vi "Fit Points to Circle.vi"(6 "Full Circle Plot":bool=TRUE, 8 "Error In":errorcluster, 9 "# Points (1000)":i32=1000, 10 "Y Array":dbl[](array[numeric]), 11 "X Array":dbl[](array[numeric])) -> (0 "Error Out":errorcluster, 3 "Fitted Circle Parameters":T1, 5 "Fitted Y Array":dbl[](array[numeric]), 7 "Fitted X Array":dbl[](array[numeric]))   [LabVIEW 2019]
uses:
  Fitted Circle Parameters.ctl
  <vilib>/Utility/error.llb/DialogType.ctl
  <vilib>/Utility/error.llb/Error Cluster From Error Code.vi
  <vilib>/ErrorRing/Error Ring.xnode
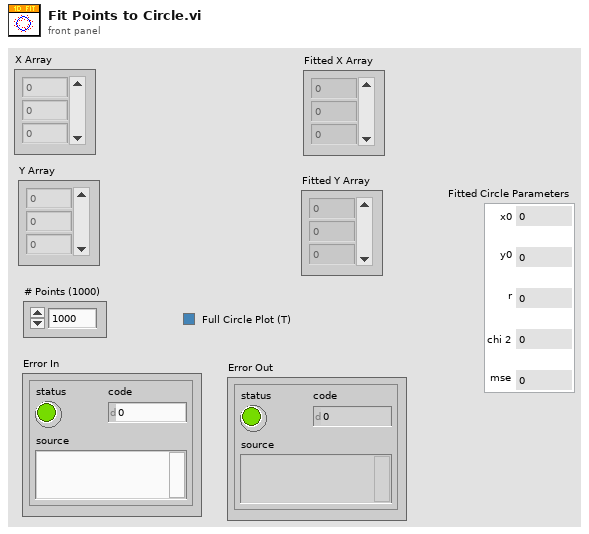
[diagram p1: front panel]
types:
  T1 = typedef "Fitted Circle Parameters.ctl" = cluster{"x0":dbl, "y0":dbl, "r":dbl, "chi 2":dbl, "mse":dbl}
  T2 = typedef "DialogType.ctl" = u16
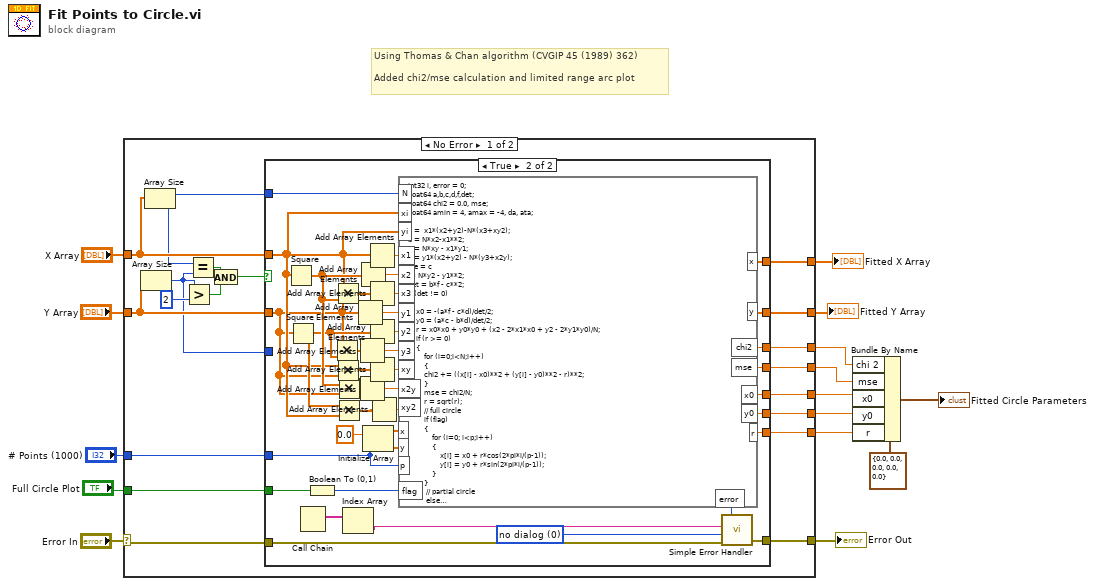
[diagram p0: block diagram]
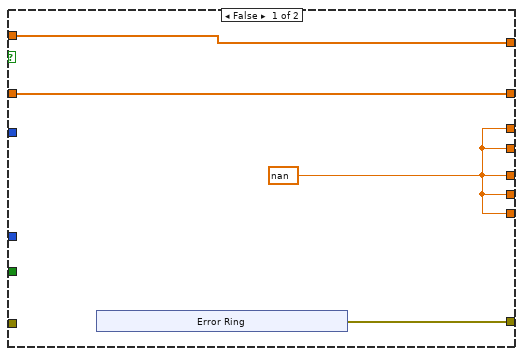
[diagram p2: hidden frame]
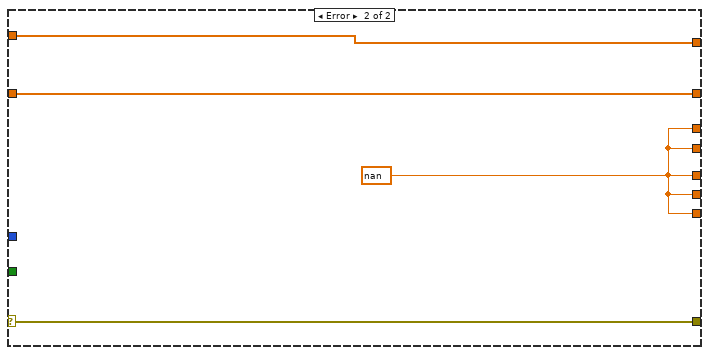
[diagram p3: hidden frame]
diagram:
  # "Using Thomas & Chan algorithm (CVGIP 45 (1989) 362)\n\nAdded chi2/mse calculation and limited range arc plot"
  n1 = case shown="No Error" "Error In" {
    selector: "Error In" -> [w20 w83]
    tunnel: "X Array" -> [w34 w82]
    tunnel: "Y Array" -> [w33 w81]
    tunnel: [w21 w83] -> w12
    tunnel: [w26 w82] -> w11
    tunnel: [w25 w81] -> w10
    tunnel: "# Points (1000)" -> [w27 _]
    tunnel: [w24 w80] -> w6
    tunnel: [w23 w80] -> w7
    tunnel: [w22 w80] -> w8
    tunnel: [w18 w80] -> w4
    tunnel: [w17 w80] -> w5
    tunnel: "Full Circle Plot" -> [w16 _]
    frame No Error {
      n2 = Array Size(array=w33) -> (size(s)=w28:i32)
      n3 = Array Size(array=w34) -> (size(s)=w19:i32)
      n4 = Greater?(x=w28, y=2) -> (0:w31:bool)
      n5 = Equal?(x=w19, y=w28) -> (x = y?=w30:bool)
      n6 = And(x=w30, y=w31) -> (x .and. y?=w29:bool)
      n7 = case shown="True" w29 {
        tunnel: w34 -> [w37 w44]
        tunnel: w33 -> [w36 w43]
        tunnel: w28 -> [_ _]
        tunnel: w27 -> [_ w49]
        tunnel: [w37 w77] -> w26
        tunnel: [w36 w76] -> w25
        tunnel: [w35 w75] -> w24
        tunnel: [w35 w74] -> w23
        tunnel: [w35 w73] -> w22
        tunnel: [w38 w56] -> w21
        tunnel: w20 -> [_ w55]
        tunnel: w19 -> [_ w50]
        tunnel: [w35 w48] -> w18
        tunnel: [w35 w47] -> w17
        tunnel: w16 -> [_ w46]
        frame False {
          w35 = nan ("x0")
          n8 = xnode "Error Ring"() -> ("error out"=w38:errorcluster)
        }
        frame True {
          w51 = T2 0 items=["no dialog", "OK message", "continue or stop message", "OK message + warnings", "continue/stop + warnings"] ("type of dialog (OK msg:1)")
          n9 = Square(x=w44) -> (x^2=w62:dbl[])
          n10 = Square(x=w43) -> (x^2=w59:dbl[])
          n11 = Call Chain() -> (call chain=w53:string[])
          n12 = Boolean To (0,1)(Boolean=w46) -> (0, 1=w45:i16)
          n13 = Multiply(x=w43, y=w59) -> (x*y=w70:dbl[])
          n14 = Multiply(x=w44, y=w62) -> (x*y=w72:dbl[])
          n15 = Multiply(x=w44, y=w43) -> (x*y=w64:dbl[])
          n16 = Multiply(x=w62, y=w43) -> (x*y=w61:dbl[])
          n17 = Multiply(x=w59, y=w44) -> (x*y=w58:dbl[])
          n18 = Index Array(array=w53) -> (element=w52:string)  [unwired: 1 in]
          n19 = Add Array Elements(numeric array=w43) -> (sum=w71:dbl)
          n20 = Add Array Elements(numeric array=w70) -> (sum=w68:dbl)
          n21 = Add Array Elements(numeric array=w61) -> (sum=w60:dbl)
          n22 = Add Array Elements(numeric array=w62) -> (sum=w65:dbl)
          n23 = Initialize Array(0.0 ("element"), w49) -> (w79:dbl[])
          n24 = Add Array Elements(numeric array=w44) -> (sum=w69:dbl)
          n25 = Add Array Elements(numeric array=w72) -> (sum=w67:dbl)
          n26 = Add Array Elements(numeric array=w59) -> (sum=w66:dbl)
          n27 = Add Array Elements(numeric array=w64) -> (sum=w63:dbl)
          n28 = Add Array Elements(numeric array=w58) -> (sum=w57:dbl)
          n29 = formula code="int32 i, error = 0;\nfloat64 a,b,c,d,f,det;\nfloat64 chi2 = 0.0, mse;\nfloat64 amin = 4, amax = -4, da, ata;\n\na =  x1*(x2+y2)-N*(x3+xy2);\nb = N*x2-x1**2;\nc = N*xy - x1*y1;\nd = y1*(x2+y2) - N*(y3+x2y);\n// e = c\nf= N*y2 - y1**2;\ndet = b*f - c**2;\nif (det != 0)\n{\n    x0 = -(a*f - c*d)/det/2;\n    y0 = (a*c - b*d)/det/2;\n    r = x0*x0 + y0*y0 + (x2 - 2*x1*x0 + y2 - 2*y1*y0)/N;\n    if (r >= 0)\n    {\n        for (i=0;i<N;i++)\n        {\n        chi2 += ((x[i] - x0)**2 + (y[i] - y0)**2 - r)**2;\n        }\n        mse = chi2/N;\n        r = sqrt(r);\n        // full circle\n        if (flag)\n        {\n            for (i=0; i<p;i++)\n            {\n                x[i] = x0 + r*cos(2*pi*i/(p-1));\n                y[i] = y0 + r*sin(2*pi*i/(p-1));\n            }\n        }\n         // partial circle\n         else\n          {\n             for (i=0; i<N;i++)\n             {\n                 ata = atan2(yi[i] - y0,xi[i] - x0);\n                 ata = (ata < 0) ? ata + 2*pi : ata;\n                 amin = (ata < amin) ? ata : amin;\n                 amax = (ata > amax) ? ata : amax;\n             }\n             da = (amax - amin)/(p - 1);\n             for (i=0; i<p;i++)\n             {\n                x[i] = x0 + r*cos(amin+ da*i);\n                y[i] = y0 + r*sin(amin+ da*i);\n             }\n          }\n       }\n    else\n        error = -23042; // radius squared is negative\n}"("x1"=w69, "x2"=w65, "x3"=w67, "y1"=w71, "y2"=w66, "y3"=w68, "xy"=w63, "x2y"=w60, "xy2"=w57, "x"=w79, "y"=w79, "N"=w50, "p"=w49, "flag"=w45, "xi"=w44, "yi"=w43) -> ("x0"=w75:dbl, "y0"=w74:dbl, "r"=w73:dbl, "x"=w77:dbl[], "y"=w76:dbl[], "error"=w54:i32, "chi2"=w48:dbl, "mse"=w47:dbl)
          n30 = call <vilib>:"Simple Error Handler.vi"("error code (no error:0)"=w54, "error source (\" \")"=w52, "type of dialog (OK msg:1)"=w51, "error in (no error)"=w55) -> ("error out"=w56:errorcluster)  [unwired: 1 in, 4 out]
        }
      }
    }
    frame Error {
      w80 = nan ("x0")
    }
  }
  "Error Out" <- w12
  "Fitted X Array" <- w11
  "Fitted Y Array" <- w10
  n31 = Bundle By Name(cluster=T1 {"x0"=0.0, "y0"=0.0, "r"=0.0, "chi 2"=0.0, "mse"=0.0} ("Fitted Circle Parameters"), "chi 2"=w4, "mse"=w5, "x0"=w6, "y0"=w7, "r"=w8) -> (→"Fitted Circle Parameters":T1)
